vi "CreateStand.vi"(0 "Stand in":refnum<class "Stand.lvclass">, 5 "error in (no error)":errorcluster, 7 "FPGA API":refnum<class "FPGA API.lvclass">, 8 "Modbus":refnum<class "ModbusSp.lvclass">, 9 "ConfigInterface":refnum<class "ConfigInterface.lvclass">, 10 "NV Addres":string="192.168.1.100", 11 "SV_Publisher":refnum<class "SV_Publisher.lvclass">, 12 "Tags":T1, 13 "Logger":refnum<class "Logger.lvclass">) -> (14 "Stand out":refnum<class "Stand.lvclass">, 19 "error out":errorcluster)   [LabVIEW 2019, in "Stand.lvclass"]
uses:
  Stand.lvclass
  C:/Users/ANENKOV_V1/Desktop/src/Device_class/Device.lvclass
  C:/Users/ANENKOV_V1/Desktop/src/Proccess_class/Proccess.lvclass
  FPGA_API_class/FPGA API.lvclass
  ConfigInterface_class/ConfigInterface.lvclass
  SV_Puplisher_class/SV_Publisher.lvclass
  Proccess_class/TAGs.ctl
  Logger_class/Logger.lvclass
  Modbus_class/ModbusSp.lvclass
  Stand.lvclass/Stand.ctl
  Proccess_class/Proccess.lvclass/Proccess.ctl
  Device_class/Device.lvclass/Device.ctl
  Valve_2DO_2DI_class/DIO.ctl
  FPGA/TypeDef/DO index.ctl
  FPGA/TypeDef/DI index.ctl
  dY_dX_Calculator/delayValue.lvclass/delayValue.ctl
  <vilib>/Utility/error.llb/Clear Errors.vi
  MessageInterface_class/MessageInterface.lvclass
  Device_class/Device.lvclass
  Proccess_class/Proccess.lvclass
  PM_Group_class/PM_Group.lvclass
  NeedleValve_class/NeedleValve.lvclass
  Valve_2DO_2DI_class/Valve_2DO_2DI.lvclass
  dY_dX_Calculator/delayValue.lvclass
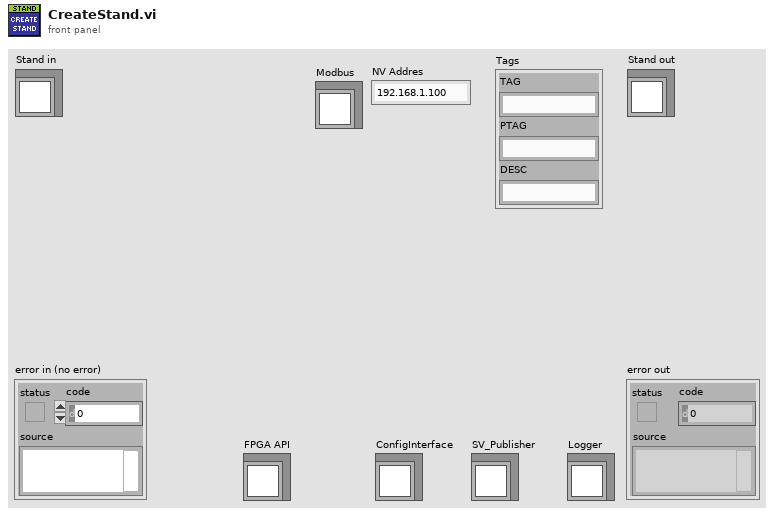
[diagram p1: front panel]
types:
  T1 = typedef "Proccess.lvclass/TAGs.ctl" = cluster{"TAG":string, "PTAG":string, "DESC":string}
  T2 = typedef "Valve_2DO_2DI.lvclass/DIO.ctl" = cluster{"DO Open":T3, "DI Open":T4, "DI Close":T4, "DO Close":T3}
  T3 = typedef "DO index.ctl" = u8
  T4 = typedef "DI index.ctl" = u8
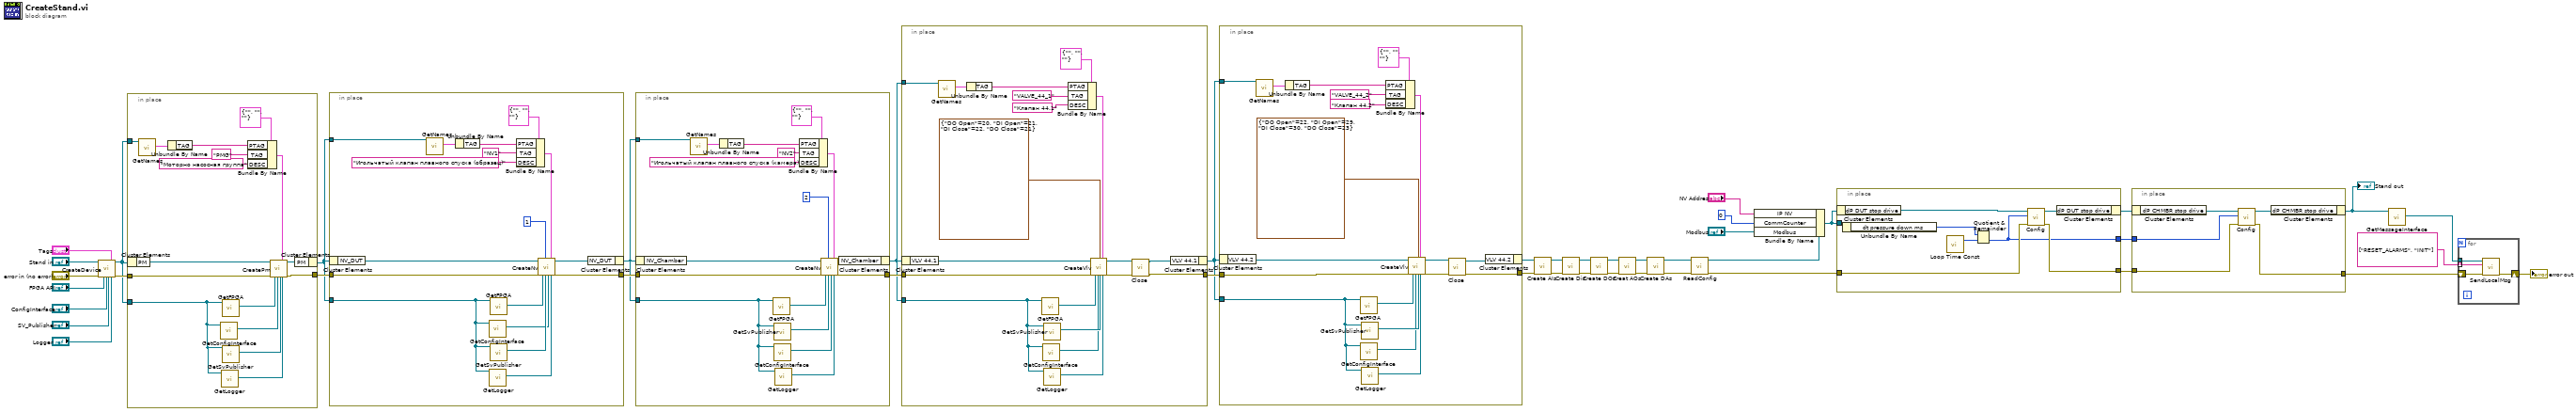
[diagram p0: block diagram]
diagram:
  n1 = call "CreateDevice.vi"("Device in"="Stand in", "error in (no error)"="error in (no error)", "FPGA API"="FPGA API", "ConfigInterface"="ConfigInterface", "SV_Publisher"="SV_Publisher", "Tags"="Tags", "Logger"="Logger") -> ("Device out"=w35:refnum<class "Stand.lvclass">, "error out"=w36:errorcluster)  [unwired: 11 in]
  n2 = in-place {
    in-place-border: w35 -> [w57]
    in-place-border: w35 -> [w48]
    in-place-border: w36 -> [w46]
    in-place-border: [w45] -> w34
    n3 = in-place-cluster #1(w35) -> ("PM"=w59:refnum<class "PM_Group.lvclass">)
    n4 = call "GetNames.vi"("Proccess in"=w57) -> ("Tags"=w54:T1)  [unwired: 10 in]
    n5 = Unbundle By Name(w54) -> ("TAG"=w53:string)
    n6 = call "GetConfigInterface.vi"("Device in"=w48) -> ("ConfigInterface"=w49:refnum<class "ConfigInterface.lvclass">)  [unwired: 10 in]
    n7 = call "GetLogger.vi"("Proccess in"=w48) -> ("Logger"=w47:refnum<class "Logger.lvclass">)  [unwired: 10 in]
    n8 = call "GetFPGA.vi"("Device in"=w48) -> ("FPGA API.lvclass"=w51:refnum<class "FPGA API.lvclass">)  [unwired: 10 in]
    n9 = call "GetSvPublisher.vi"("Device in"=w48) -> ("SV_Publisher.lvclass"=w50:refnum<class "SV_Publisher.lvclass">)  [unwired: 10 in]
    n10 = Bundle By Name(cluster=T1 {"TAG"="", "PTAG"="", "DESC"=""} ("Tags"), "PTAG"=w53, "TAG"="PMG", "DESC"="Моторно насосная группа") -> (w55:T1)
    n11 = call "CreatePm.vi"("PM_Group in"=w59, "error in (no error)"=w46, "FPGA API"=w51, "ConfigInterface"=w49, "SV_Publisher"=w50, "Tags"=w55, "Logger"=w47) -> ("PM_Group out"=w58:refnum<class "PM_Group.lvclass">, "error out"=w45:errorcluster)  [unwired: 11 in]
    n12 = in-place-cluster #1("PM"=w58) -> (w33:refnum<class "Stand.lvclass">)
  }
  n13 = in-place {
    in-place-border: w33 -> [w74]
    in-place-border: w33 -> [w65]
    in-place-border: w34 -> [w63]
    in-place-border: [w62] -> w32
    n14 = in-place-cluster #2(w33) -> ("NV_DUT"=w76:refnum<class "NeedleValve.lvclass">)
    n15 = call "GetNames.vi"("Proccess in"=w74) -> ("Tags"=w71:T1)  [unwired: 10 in]
    n16 = Unbundle By Name(w71) -> ("TAG"=w70:string)
    n17 = call "GetConfigInterface.vi"("Device in"=w65) -> ("ConfigInterface"=w66:refnum<class "ConfigInterface.lvclass">)  [unwired: 10 in]
    n18 = call "GetLogger.vi"("Proccess in"=w65) -> ("Logger"=w64:refnum<class "Logger.lvclass">)  [unwired: 10 in]
    n19 = call "GetFPGA.vi"("Device in"=w65) -> ("FPGA API.lvclass"=w68:refnum<class "FPGA API.lvclass">)  [unwired: 10 in]
    n20 = call "GetSvPublisher.vi"("Device in"=w65) -> ("SV_Publisher.lvclass"=w67:refnum<class "SV_Publisher.lvclass">)  [unwired: 10 in]
    n21 = Bundle By Name(cluster=T1 {"TAG"="", "PTAG"="", "DESC"=""} ("Tags"), "PTAG"=w70, "TAG"="NV1", "DESC"="Игольчатый клапан плавного спуска (образец)") -> (w72:T1)
    n22 = call "CreateNv.vi"("NeedleValve in"=w76, "error in (no error)"=w63, "FPGA API"=w68, "addres"=u16 1, "SV_Publisher"=w67, "ConfigInterface"=w66, "Tags"=w72, "Logger"=w64) -> ("NeedleValve out"=w75:refnum<class "NeedleValve.lvclass">, "error out"=w62:errorcluster)  [unwired: 10 in]
    n23 = in-place-cluster #2("NV_DUT"=w75) -> (w31:refnum<class "Stand.lvclass">)
  }
  n24 = in-place {
    in-place-border: w31 -> [w91]
    in-place-border: w31 -> [w82]
    in-place-border: w32 -> [w80]
    in-place-border: [w79] -> w30
    n25 = in-place-cluster #3(w31) -> ("NV_Chamber"=w93:refnum<class "NeedleValve.lvclass">)
    n26 = call "GetNames.vi"("Proccess in"=w91) -> ("Tags"=w88:T1)  [unwired: 10 in]
    n27 = Unbundle By Name(w88) -> ("TAG"=w87:string)
    n28 = call "GetFPGA.vi"("Device in"=w82) -> ("FPGA API.lvclass"=w85:refnum<class "FPGA API.lvclass">)  [unwired: 10 in]
    n29 = call "GetConfigInterface.vi"("Device in"=w82) -> ("ConfigInterface"=w83:refnum<class "ConfigInterface.lvclass">)  [unwired: 10 in]
    n30 = call "GetSvPublisher.vi"("Device in"=w82) -> ("SV_Publisher.lvclass"=w84:refnum<class "SV_Publisher.lvclass">)  [unwired: 10 in]
    n31 = call "GetLogger.vi"("Proccess in"=w82) -> ("Logger"=w81:refnum<class "Logger.lvclass">)  [unwired: 10 in]
    n32 = Bundle By Name(cluster=T1 {"TAG"="", "PTAG"="", "DESC"=""} ("Tags"), "PTAG"=w87, "TAG"="NV2", "DESC"="Игольчатый клапан плавного спуска (камера)") -> (w89:T1)
    n33 = call "CreateNv.vi"("NeedleValve in"=w93, "error in (no error)"=w80, "FPGA API"=w85, "addres"=u16 2, "SV_Publisher"=w84, "ConfigInterface"=w83, "Tags"=w89, "Logger"=w81) -> ("NeedleValve out"=w92:refnum<class "NeedleValve.lvclass">, "error out"=w79:errorcluster)  [unwired: 10 in]
    n34 = in-place-cluster #3("NV_Chamber"=w92) -> (w29:refnum<class "Stand.lvclass">)
  }
  n35 = in-place {
    in-place-border: w29 -> [w111]
    in-place-border: w29 -> [w102]
    in-place-border: w30 -> [w100]
    in-place-border: [w94] -> w28
    n36 = in-place-cluster #4(w29) -> ("VLV 44.1"=w112:refnum<class "Valve_2DO_2DI.lvclass">)
    n37 = call "GetNames.vi"("Proccess in"=w111) -> ("Tags"=w108:T1)  [unwired: 10 in]
    n38 = Unbundle By Name(w108) -> ("TAG"=w107:string)
    n39 = call "GetFPGA.vi"("Device in"=w102) -> ("FPGA API.lvclass"=w105:refnum<class "FPGA API.lvclass">)  [unwired: 10 in]
    n40 = call "GetConfigInterface.vi"("Device in"=w102) -> ("ConfigInterface"=w103:refnum<class "ConfigInterface.lvclass">)  [unwired: 10 in]
    n41 = call "GetSvPublisher.vi"("Device in"=w102) -> ("SV_Publisher.lvclass"=w104:refnum<class "SV_Publisher.lvclass">)  [unwired: 10 in]
    n42 = call "GetLogger.vi"("Proccess in"=w102) -> ("Logger"=w101:refnum<class "Logger.lvclass">)  [unwired: 10 in]
    n43 = Bundle By Name(cluster=T1 {"TAG"="", "PTAG"="", "DESC"=""} ("Tags"), "PTAG"=w107, "TAG"="VALVE_44_1", "DESC"="Клапан 44.1" ("TAG")) -> (w109:T1)
    n44 = call "CreateVlv.vi"("Pump_1AI_1DO_2DI in"=w112, "error in (no error)"=w100, "FPGA API"=w105, "ConfigInterface"=w103, "DIO"=T2 {"DO Open"=20, "DI Open"=21, "DI Close"=22, "DO Close"=21}, "SV_Publisher"=w104, "Tags"=w109, "Logger"=w101) -> ("Pump_1AI_1DO_2DI out"=w97:refnum<class "Valve_2DO_2DI.lvclass">, "error out"=w95:errorcluster)  [unwired: 10 in]
    n45 = call "Close.vi"("error in (no error)"=w95, "Pump_1AI_1DO_2DI in"=w97) -> ("error out"=w94:errorcluster, "Pump_1AI_1DO_2DI out"=w96:refnum<class "Valve_2DO_2DI.lvclass">)  [unwired: 8 in]
    n46 = in-place-cluster #4("VLV 44.1"=w96) -> (w27:refnum<class "Stand.lvclass">)
  }
  n47 = in-place {
    in-place-border: w27 -> [w130]
    in-place-border: w27 -> [w121]
    in-place-border: w28 -> [w119]
    in-place-border: [w113] -> w26
    n48 = in-place-cluster #5(w27) -> ("VLV 44.2"=w131:refnum<class "Valve_2DO_2DI.lvclass">)
    n49 = call "GetNames.vi"("Proccess in"=w130) -> ("Tags"=w127:T1)  [unwired: 10 in]
    n50 = Unbundle By Name(w127) -> ("TAG"=w126:string)
    n51 = call "GetFPGA.vi"("Device in"=w121) -> ("FPGA API.lvclass"=w124:refnum<class "FPGA API.lvclass">)  [unwired: 10 in]
    n52 = call "GetConfigInterface.vi"("Device in"=w121) -> ("ConfigInterface"=w122:refnum<class "ConfigInterface.lvclass">)  [unwired: 10 in]
    n53 = call "GetSvPublisher.vi"("Device in"=w121) -> ("SV_Publisher.lvclass"=w123:refnum<class "SV_Publisher.lvclass">)  [unwired: 10 in]
    n54 = call "GetLogger.vi"("Proccess in"=w121) -> ("Logger"=w120:refnum<class "Logger.lvclass">)  [unwired: 10 in]
    n55 = Bundle By Name(cluster=T1 {"TAG"="", "PTAG"="", "DESC"=""} ("Tags"), "PTAG"=w126, "TAG"="VALVE_44_2", "DESC"="Клапан 44.2" ("TAG")) -> (w128:T1)
    n56 = call "CreateVlv.vi"("Pump_1AI_1DO_2DI in"=w131, "error in (no error)"=w119, "FPGA API"=w124, "ConfigInterface"=w122, "DIO"=T2 {"DO Open"=22, "DI Open"=29, "DI Close"=30, "DO Close"=23}, "SV_Publisher"=w123, "Tags"=w128, "Logger"=w120) -> ("Pump_1AI_1DO_2DI out"=w116:refnum<class "Valve_2DO_2DI.lvclass">, "error out"=w115:errorcluster)  [unwired: 10 in]
    n57 = call "Close.vi"("error in (no error)"=w115, "Pump_1AI_1DO_2DI in"=w116) -> ("error out"=w113:errorcluster, "Pump_1AI_1DO_2DI out"=w114:refnum<class "Valve_2DO_2DI.lvclass">)  [unwired: 8 in]
    n58 = in-place-cluster #5("VLV 44.2"=w114) -> (w25:refnum<class "Stand.lvclass">)
  }
  n59 = call "Create AIs.vi"("reference in"=w25, "error in (no error)"=w26) -> ("reference out"=w24:refnum<class "Stand.lvclass">, "error out"=w23:errorcluster)  [unwired: 12 in]
  n60 = call "Create Dis.vi"("reference in"=w24, "error in (no error)"=w23) -> ("reference out"=w20:refnum<class "Stand.lvclass">, "error out"=w19:errorcluster)  [unwired: 12 in]
  n61 = call "Create DOs.vi"("reference in"=w20, "error in (no error)"=w19) -> ("reference out"=w17:refnum<class "Stand.lvclass">, "error out"=w18:errorcluster)  [unwired: 12 in]
  n62 = call "Creat AOs.vi"("reference in"=w17, "error in (no error)"=w18) -> ("reference out"=w15:refnum<class "Stand.lvclass">, "error out"=w16:errorcluster)  [unwired: 12 in]
  n63 = call "Create DAs.vi"("reference in"=w15, "error in (no error)"=w16) -> ("reference out"=w13:refnum<class "Stand.lvclass">, "error out"=w14:errorcluster)  [unwired: 12 in]
  n64 = call-dynamic "ReadConfig.vi"("reference in"=w13, "error in (no error)"=w14) -> ("reference out"=w2:refnum<class "Stand.lvclass">, "error out"=w1:errorcluster)  [unwired: 12 in]
  n65 = Bundle By Name(cluster=w2, "IP NV"="NV Addres", "CommCounter"=u64 0, "Modbus"="Modbus") -> (w5:refnum<class "Stand.lvclass">)
  n66 = in-place {
    in-place-border: w1 -> [w137]
    in-place-border: [w135] -> w10
    in-place-border: [w134] -> w9
    in-place-border: w5 -> [w133]
    n67 = in-place-cluster #6(w5) -> ("dP DUT stop drive"=w139:refnum<class "delayValue.lvclass">)
    n68 = Unbundle By Name(w133) -> ("dt pressure down ms"=w132:i32)
    n69 = call "Loop Time Const.vi"() -> ("loop time ms"=w136:i64)  [unwired: 3 in]
    n70 = Quotient & Remainder(x=w132, y=w136) -> (floor(x/y)=w134:i64)  [unwired: 1 out]
    n71 = call "Config.vi"("error in (no error)"=w137, "size (10)"=w134, "dY_dX_Calculator in"=w139) -> ("error out"=w135:errorcluster, "dY_dX_Calculator out"=w138:refnum<class "delayValue.lvclass">)  [unwired: 7 in]
    n72 = in-place-cluster #6("dP DUT stop drive"=w138) -> (w11:refnum<class "Stand.lvclass">)
  }
  n73 = in-place {
    in-place-border: w10 -> [w142]
    in-place-border: [w140] -> w3
    in-place-border: w9 -> [w141]
    n74 = in-place-cluster #7(w11) -> ("dP CHMBR stop drive"=w144:refnum<class "delayValue.lvclass">)
    n75 = call "Config.vi"("error in (no error)"=w142, "size (10)"=w141, "dY_dX_Calculator in"=w144) -> ("error out"=w140:errorcluster, "dY_dX_Calculator out"=w143:refnum<class "delayValue.lvclass">)  [unwired: 7 in]
    n76 = in-place-cluster #7("dP CHMBR stop drive"=w143) -> (w4:refnum<class "Stand.lvclass">)
  }
  "Stand out" <- w4
  n77 = call "GetMessageInterface.vi"("Device in"=w4) -> ("MessageInterface"=w8:refnum<class "MessageInterface.lvclass">)  [unwired: 10 in]
  n78 = for {
    tunnel: w8 -> [w148]
    tunnel: string[] ["RESET_ALARMS", "INIT"] ("name") -> [w147] mode=indexing
    shift-right: [w146] -> w6
    shift-left: w3 -> [w145]
    n79 = call-dynamic "SendLocalMsg.vi"("reference in"=w148, "name"=w147, "error in (no error)"=w145) -> ("error out"=w146:errorcluster)  [unwired: 10 in, 2 out]
  }
  "error out" <- w6
